vi "Controls.vi"(11 "Close":bool) -> ()   [LabVIEW 2014]
panel:
  # "Joystick Mapping\n\nJoysticks: j1, j2, j3\n\nj1:\n     Y-Axis => Y-Axis Tank Drive Left\n     X-Axis => X-Axis Tank Drive Left\n\nj2:\n     Y-Axis => Y-Axis Tank Drive Right\n     X-Axis => X-Axis Tank Drive Right\n     Y + X-Axis => Arcade Drive\n     Trigger => Retract Claw, Extend when Released\n\nj3:\n     Y-Axis => Up/Down Arm\n     Button 7 => Left 2CAN Up\n     Button 6 => Left 2CAN Down\n     Button 10 => Right 2CAN Up\n     Button 11 => Right 2CAN Down\n     Button 2 => Claw Open, Closed when Released"
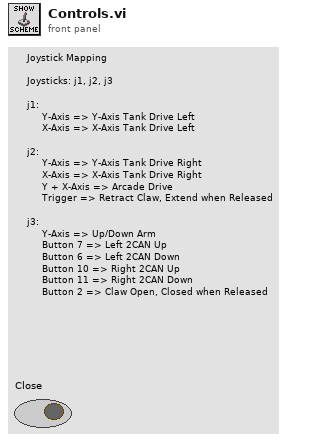
[diagram p1: front panel]
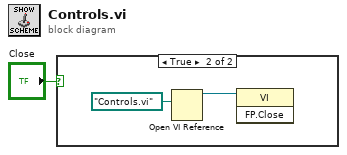
[diagram p0: block diagram]
diagram:
  n1 = case shown="True" "Close" {
    frame False {
    }
    frame True {
      n2 = Open VI Reference(vi path=path "Controls.vi") -> (vi reference=w3:refnum<vi>)  [unwired: 5 in, 1 out]
      n3 = invoke class="VI" method="FP.Close"(reference=w3) -> ()  [unwired: 2 in, 3 out]
    }
  }
